vi "Read Arm Operation.vi"(8 "Command Info":T2) -> (0 "Command Info":T2, 1 "SubSystem Data":T1, 2 "Command Timing":cluster{"Start Time (ms)":u32, "Iterations":i32})   [LabVIEW 2023]
doc: "This returns the most recently scheduled command. This doesn't indicate whether the command finished and is running the default command."
uses:
  <vilib>/Rock Robotics/WPI/Framework/Command Status Info.ctl
  <vilib>/Rock Robotics/WPI/Framework/Completion Status.ctl
  <vilib>/Rock Robotics/WPI/Framework/Completion Notifier.ctl
  Implementation/Arm Setpoints.ctl
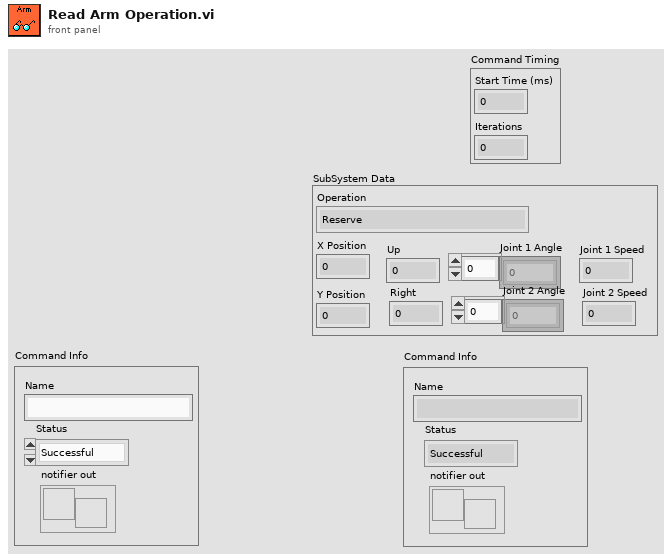
[diagram p1: front panel]
types:
  T1 = typedef "Arm Setpoints.ctl" = cluster{"Operation":enum16{"Reserve", "Read Current", "Immediate", "Move to position", "Adjust position", "Cube extend", "Cone extend", "Rotate Arm Joints", "Maintain Angle", "Retract", "Go_to_next"}, "X Position":dbl, "Y Position":dbl, "Up":dbl, "Right":dbl, "Joint 1 Angle":dbl[], "Joint 2 Angle":dbl[], "Joint 1 Speed":dbl, "Joint 2 Speed":dbl}
  T2 = typedef "Command Status Info.ctl" = cluster{"Name":string, "Status":T3, "notifier out":T4}
  T3 = typedef "Completion Status.ctl" = enum16{"Successful", "Aborted", "Incomplete"}
  T4 = typedef "Completion Notifier.ctl" = refnum<notifier>
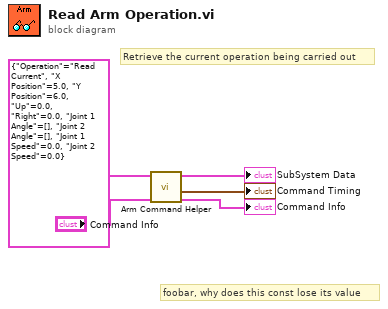
[diagram p0: block diagram]
diagram:
  # "foobar, why does this const lose its value"
  # "Retrieve the current operation being carried out"
  n1 = call "Arm Command Helper.vi"("Command Info In"="Command Info", "SubSystem Data"=T1 {"Operation"=enum."Read Current", "X Position"=5.0, "Y Position"=6.0, "Up"=0.0, "Right"=0.0, "Joint 1 Angle"=[], "Joint 2 Angle"=[], "Joint 1 Speed"=0.0, "Joint 2 Speed"=0.0}) -> ("Command Info Out"=→"Command Info":T2, "Command Timing"=→"Command Timing":cluster{"Start Time (ms)":u32, "Iterations":i32}, "SubSystem Data"=→"SubSystem Data":T1)  [unwired: 7 in]
